vi "temperature-t.vi"() -> ()   [LabVIEW 2016]
uses:
  file write.vi
  <vilib>/Utility/file.llb/Write To Spreadsheet File (DBL).vi
panel:
  out "C":dbl
  out "current temperature":dbl(slide) scale=-200.0..200.0
  out "time-temperature Graph":cluster{u32[], dbl[]}(graph)
  in  "Temperatuer Address":string="9"
  out "测量次数":i32
  out "当前时间":string
  in  "stop":bool
  in  "采样间隔/ms":u32=1000
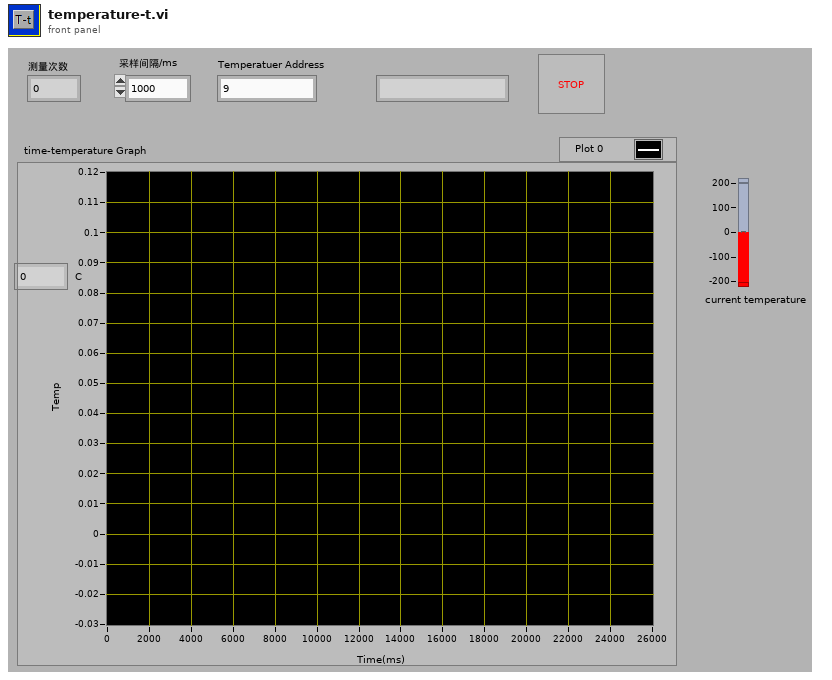
[diagram p1: front panel]
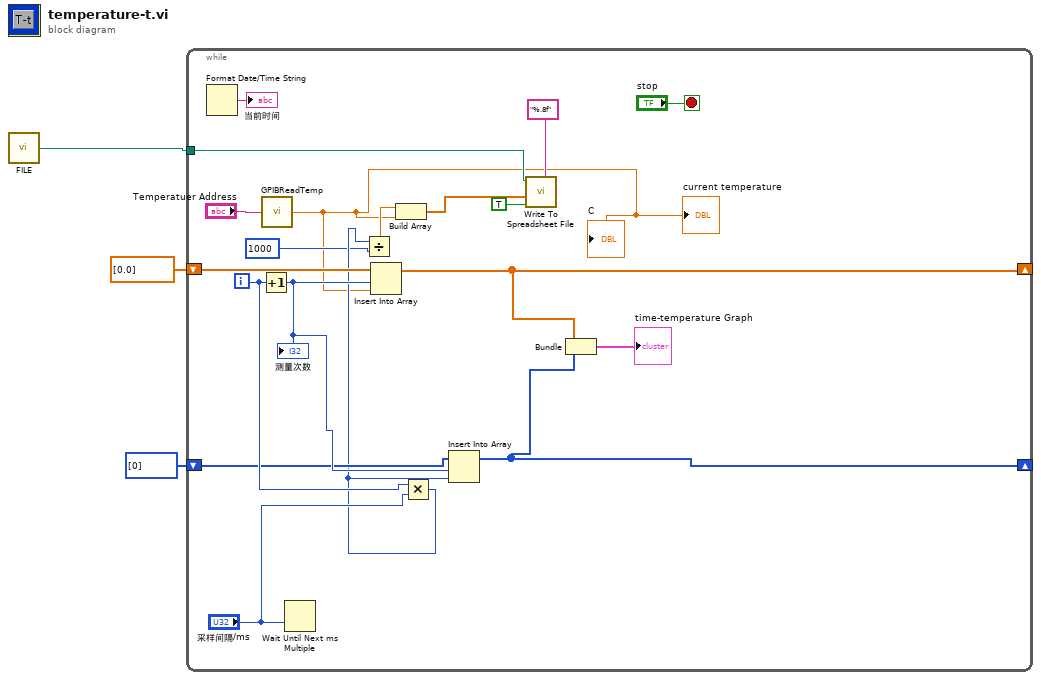
[diagram p0: block diagram]
diagram:
  n1 = call-poly "FILE.vi"() -> ("file path output"=w1:path)  [unwired: 2 in]
  n2 = while {
    shift-left: dbl[] [0.0] -> [w21]
    shift-right: [w8] -> _
    shift-right: [w12] -> _
    shift-left: u32[] [0] -> [w10]
    tunnel: w1 -> [w9]
    i -> [w13]
    stop <- "stop" stop-if-true
    n3 = Format Date/Time String() -> (date/time string=→"当前时间":string)  [unwired: 3 in]
    n4 = Increment(x=w13) -> (x+1=w11:i32)
    "测量次数" <- w11
    n5 = call "GPIBReadTemp.vi"("GPIB Address"="Temperatuer Address") -> ("Temp"=w4:dbl)
    "current temperature" <- w4
    "C" <- w4
    n6 = Wait Until Next ms Multiple(millisecond multiple="采样间隔/ms") -> ()  [unwired: 1 out]
    n7 = Insert Into Array(array=w21, index=w11, new element=w4) -> (w8:dbl[])
    n8 = Multiply(x=w13, y="采样间隔/ms") -> (x*y=w7:u32)
    n9 = Divide(x=w7, y=1000) -> (x/y=w5:dbl)
    n10 = Build Array(w5, w4) -> (w16:dbl[])
    n11 = Insert Into Array(array=w10, index=w11, new element=w7) -> (w12:u32[])
    n12 = call-poly <vilib>:"Write To Spreadsheet File.vi"("format (%.3f)"="%.8f", "append to file? (new file:F)"=TRUE, "1D data"=w16, "file path (dialog if empty)"=w9) -> ()  [unwired: 4 in, 1 out]
    n13 = Bundle(w12, w8) -> (→"time-temperature Graph":cluster{u32[], dbl[]})  [unwired: 1 in]
  }
